vi "Delivery - single appender.vi"(8 "error in (no error)":errorcluster) -> (0 "error out":errorcluster)   [LabVIEW 2026, in "Tests.lvlib"]
doc: "Integration test (Caraya). Verifies a statement logged through the Logger reaches a single registered appender. Launches a manager with the default file disabled and a queue-mode relay capture probe (Open Test Mgr), logs one INFO statement, dequeues from the capture queue with a timeout, and asserts it was delivered and its message matches. Tears down with Close Test Mgr regardless of assertion outcome (SRS-LMBR-019). Uses the manager fixture; no temp root needed.\n\nImplements LMBR-T-029 -> SRS-019. Assert-level IDs: Test-ID-Assert-Checklist.md."
uses:
  Tests.lvlib
  src/TypeDefs/Severity.ctl
  <vilib>/addons/_JKI Toolkits/Caraya/classes/Assert/Assert False.vi
  <vilib>/addons/_JKI Toolkits/Caraya/classes/Assert/Assert Equal Value_Variant.vi
  <vilib>/addons/_JKI Toolkits/Caraya/classes/Test/Test.lvclass
  src/Lumberjack.lvlib
  src/Public/Logger.lvclass/Logger.lvclass
  <vilib>/addons/_JKI Toolkits/Caraya/classes/Assert/Assert.lvclass
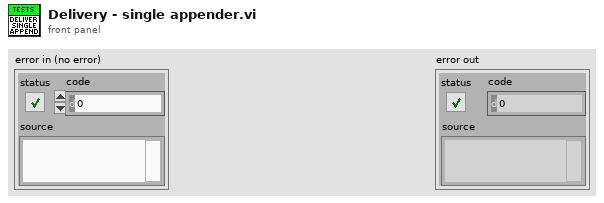
[diagram p1: front panel]
types:
  T1 = typedef "Lumberjack.lvlib/Severity.ctl" = enum16{"OFF", "FATAL", "ERROR", "WARN", "INFO", "DEBUG", "TRACE", "ALL"}
  T2 = typedef "Lumberjack.lvlib/Statement.ctl" = cluster{"timestamp":timestamp, "level":T1, "sourceTag":string, "originVI":string, "message":string}
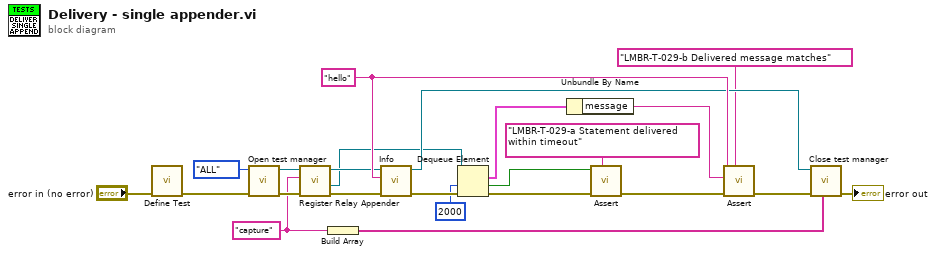
[diagram p0: block diagram]
diagram:
  w3 = "capture" ("id in")
  w13 = "hello" ("message")
  n1 = call <vilib>:"Define Test.vi"("error in (no error)"="error in (no error)") -> ("error out"=w22:errorcluster)  [unwired: 9 in, 1 out]
  n2 = call "Open test manager.vi"("error in (no error)"=w22, "globalThreshold"=Severity."ALL") -> ("error out"=w7:errorcluster, "Logger out"=w8:refnum<class "Logger.lvclass">)  [unwired: 8 in]
  n3 = call "Register Relay Appender.vi"("error in (no error)"=w7, "id in"=w3, "Logger in"=w8) -> ("error out"=w5:errorcluster, "relayQueue"=w4:refnum<queue>, "Logger out"=w6:refnum<class "Logger.lvclass">)  [unwired: 5 in, 1 out]
  n4 = Build Array(w3) -> (w1:string[])
  n5 = call "Info.vi"("error in (no error)"=w5, "message"=w13, "Logger in"=w6) -> ("error out"=w20:errorcluster, "Logger out"=w11:refnum<class "Logger.lvclass">)  [unwired: 7 in]
  n6 = Dequeue Element(queue=w4, timeout in ms (-1)=2000, error in (no error)=w20) -> (element=w15:T2, timed out?=w17:bool, error out=w18:errorcluster)  [unwired: 1 out]
  n7 = Unbundle By Name(w15) -> ("message"=w14:string)
  n8 = call-poly <vilib>:"Assert.vi"("Label"="LMBR-T-029-a Statement delivered within timeout", "error in (no error)"=w18, "False?"=w17) -> ("error out"=w16:errorcluster)  [unwired: 7 in, 1 out]
  n9 = call-poly <vilib>:"Assert.vi"("Label"="LMBR-T-029-b Delivered message matches", "error in (no error)"=w16, "Actual"=w14, "Expected"=w13) -> ("error out"=w12:errorcluster)  [unwired: 6 in, 1 out]
  n10 = call "Close test manager.vi"("queueIDList"=w1, "error in (no error)"=w12, "Logger in"=w11) -> ("error out"=→"error out":errorcluster)  [unwired: 6 in]
